vi "Ref.vi"() -> ()   [LabVIEW 2017]
uses:
  <vilib>/userdefined/High Color/IMAQdx.ctl
  <vilib>/myRIO/Common/Instrument Driver Framework/myRIO v1.0/UART/vis/myRIO v1.0 Close UART.vi
  LABVIEW2/colum_element.vi
  <vilib>/myRIO/Common/Instrument Driver Framework/Utilities/vis/FPGA Ref Manager.vi
  <vilib>/myRIO/Common/Instrument Driver Framework/myRIO v1.0/myRIO v1.0 Reset FPGA.vi
  <vilib>/myRIO/Common/Instrument Driver Framework/myRIO v1.0/IRQ/vis/myRIO v1.0 IRQ Info FGV.vi
  <vilib>/myRIO/Common/Instrument Driver Framework/myRIO v1.0/IRQ/vis/myRIO v1.0 Timer IRQ Info FGV.vi
  <vilib>/myRIO/Common/Instrument Driver Framework/myRIO v1.0/IRQ/vis/myRIO v1.0 ISR Agent.vi
  <vilib>/vision/driver/NI_Vision_Acquisition_Software.lvlib
  <vilib>/myRIO/Instrument Drivers/Utilities/Utilities.lvlib
  <vilib>/vision/NI_Vision_Development_Module.lvlib
panel:
  out "Numeric":i32
  out "Column_VALUE":i32
  out "Image Pixels (U8)":u8[][](array[numeric])
  in  "Optional Rectangle":i32[](array[numeric])=[0, 0, 640, 480]
  out "Threshold Image":T1(plugin-control)
  in  "Manual":cluster{sgl, sgl}(slide)={100.0, 255.0} caption="Threshold Range" scale=0.0..255.0
  in  "Stop":bool
  out "Image Preview":T1(plugin-control)
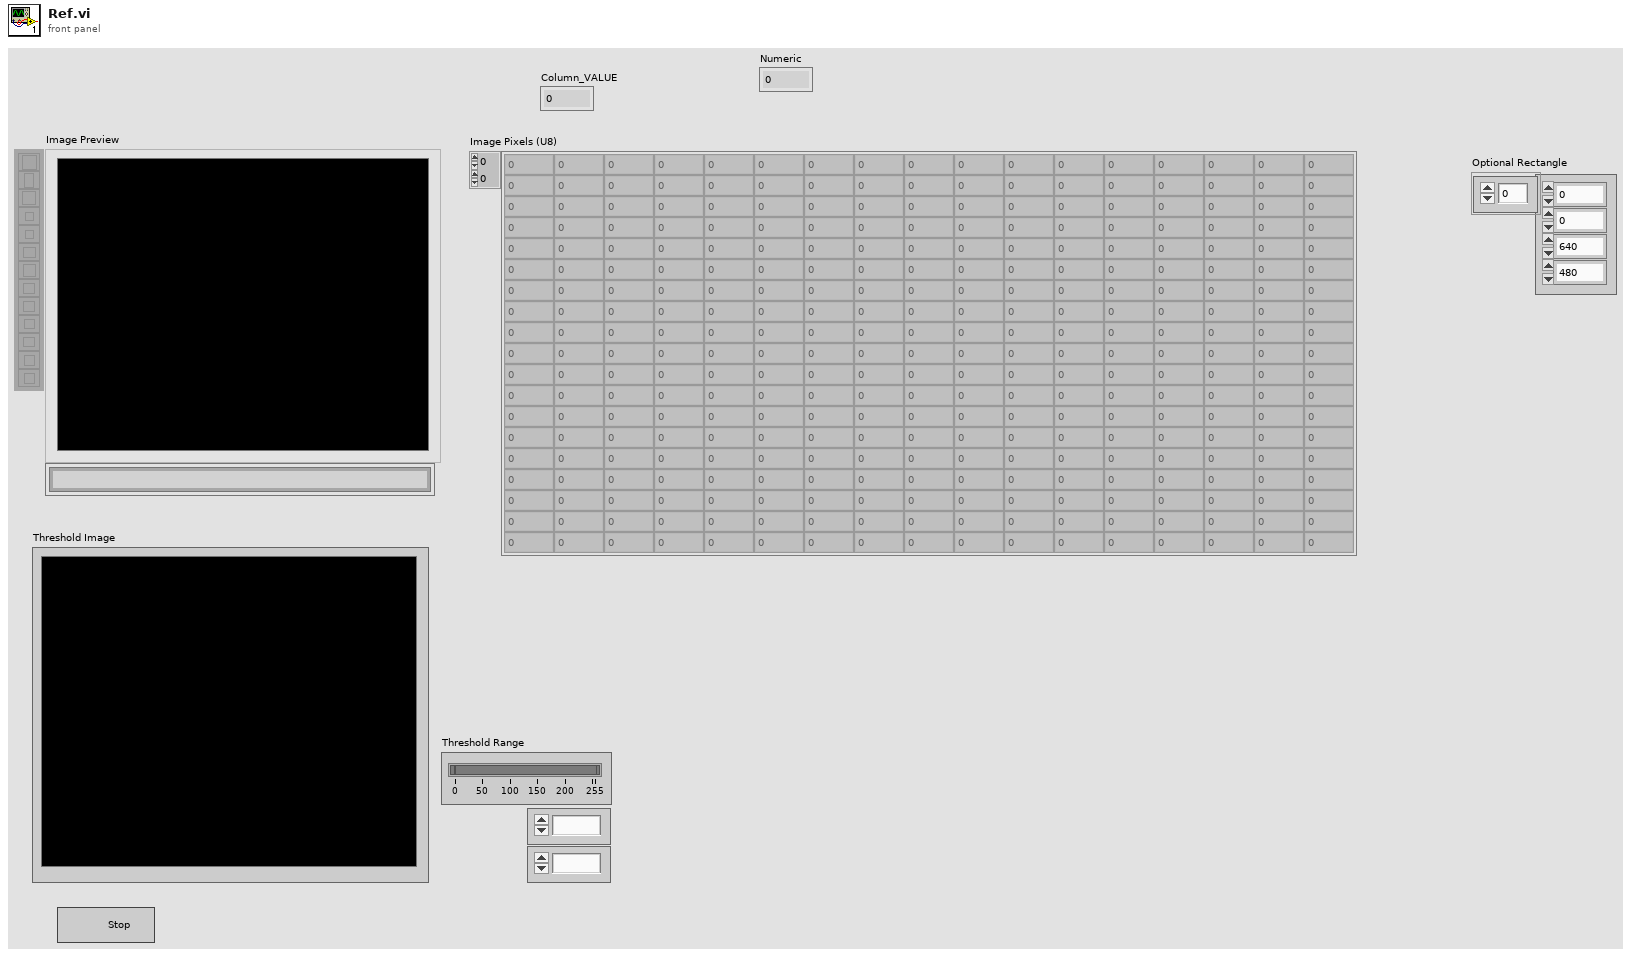
[diagram p1: front panel]
types:
  T1 = typedef "IMAQ Image.ctl" = refnum<image>
  T2 = typedef "IMAQdx.ctl" = refnum<k21>
  T3 = typedef "Image Type" = u32
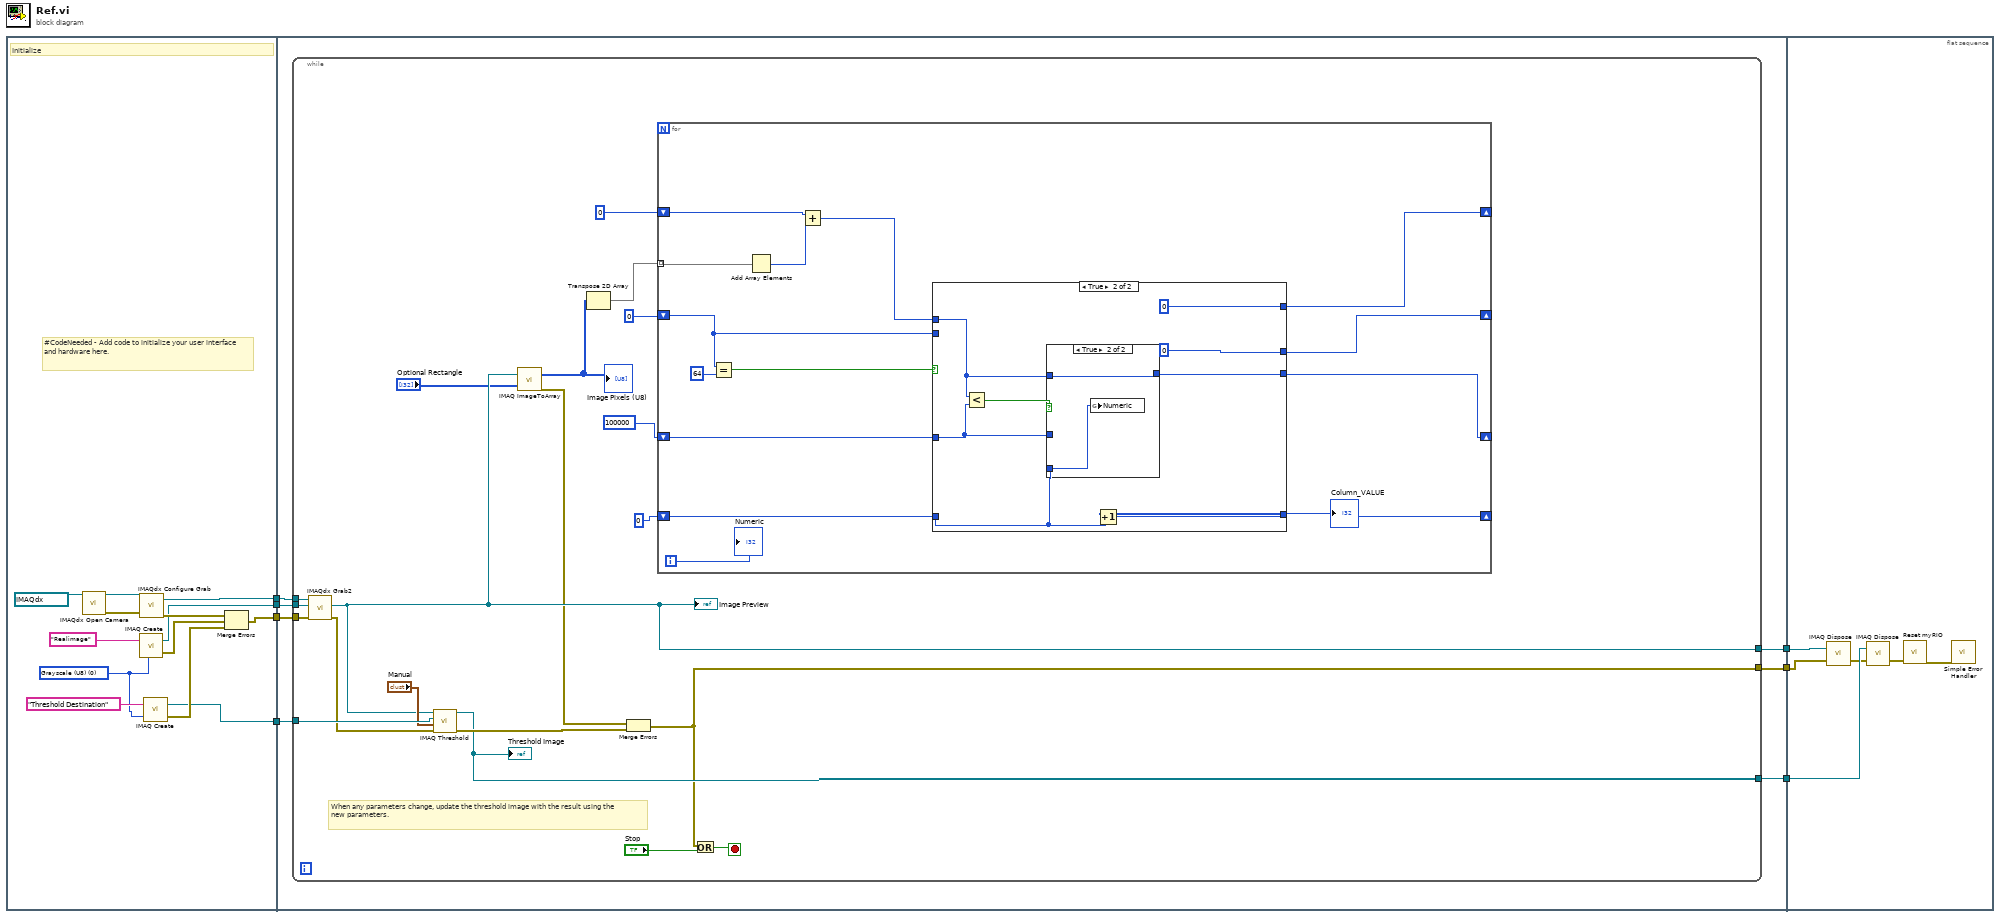
[diagram p0: block diagram]
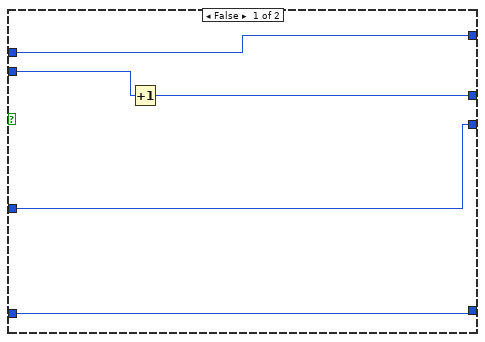
[diagram p2: hidden frame]
diagram:
  n1 = flat-sequence {
    tunnel: [w14] -> w7
    tunnel: [w13] -> w6
    tunnel: [w12] -> w5
    tunnel: [w8] -> w2
    tunnel: w7 -> [w27]
    tunnel: w6 -> [w26]
    tunnel: w5 -> [w25]
    tunnel: [w24] -> w4
    tunnel: [w23] -> w3
    tunnel: w2 -> [w22]
    tunnel: [w21] -> w1
    tunnel: w4 -> [w83]
    tunnel: w3 -> [w82]
    tunnel: w1 -> [w79]
    frame #0 {
      w10 = T3 0 items=["Grayscale (U8)", "Grayscale (I16)", "Grayscale (SGL)", "Complex (CSG)", "RGB (U32)", "HSL (U32)", "RGB (U64)", "Grayscale (U16)"] ("Image Type")
      # "#CodeNeeded - Add code to initialize your user interface and hardware here."
      # "Initialize"
      n2 = call <vilib>:"IMAQdx Open Camera.vi"("Session In"=T2 "cam0") -> ("error out"=w19:errorcluster, "Session Out"=w20:T2)  [unwired: 9 in]
      n3 = call "IMAQ Create"("Image Name"="Realimage", "Image Type"=w10) -> ("New Image"=w13:T1, "error out"=w16:errorcluster)  [unwired: 3 in]
      n4 = call <vilib>:"IMAQdx Configure Grab.vi"("error in"=w19, "Session In"=w20) -> ("error out"=w15:errorcluster, "Session Out"=w12:T2)  [unwired: 8 in]
      n5 = call "IMAQ Create"("Image Name"="Threshold Destination", "Image Type"=w10) -> ("New Image"=w8:T1, "error out"=w9:errorcluster)  [unwired: 3 in]
      n6 = Merge Errors(w15, w16, w9) -> (w14:errorcluster)
    }
    frame #1 {
      n7 = while {
        tunnel: w27 -> [w47]
        tunnel: w26 -> [w46]
        tunnel: w25 -> [w45]
        tunnel: [w35] -> w23
        tunnel: [w37] -> w24
        tunnel: w22 -> [w44]
        tunnel: [w38] -> w21
        stop <- w42 stop-if-true
        # "When any parameters change, update the threshold image with the result using the new parameters."
        n8 = call <vilib>:"IMAQdx Grab2.vi"("error in"=w47, "Image In"=w46, "Session In"=w45) -> ("error out"=w41:errorcluster, "Image Out"=w37:T1)  [unwired: 5 in, 2 out]
        "Image Preview" <- w37
        n9 = call "IMAQ Threshold"("error in (no error)"=w41, "Range"="Manual", "Image Dst"=w44, "Image Src"=w37) -> ("error out"=w40:errorcluster, "Image Dst Out"=w38:T1)  [unwired: 6 in]
        "Threshold Image" <- w38
        n10 = call "IMAQ ImageToArray"("Optional Rectangle"="Optional Rectangle", "Image"=w37) -> ("error out"=w34:errorcluster, "Image Pixels (U8)"=w33:u8[][])  [unwired: 2 in, 3 out]
        "Image Pixels (U8)" <- w33
        n11 = Transpose 2D Array(2D array=w33) -> (transposed array=w32:u8[][])
        n12 = Merge Errors(w34, w40) -> (w35:errorcluster)
        n13 = for {
          tunnel: w32 -> [w61] mode=indexing
          shift-right: [w55] -> _
          shift-left: 0 -> [w56]
          shift-right: [w51] -> _
          shift-left: 0 -> [w59]
          shift-right: [w53] -> _
          shift-left: 0 -> [w54]
          shift-right: [w48] -> _
          shift-left: 100000 -> [w49]
          i -> [w50]
          n14 = Equal?(x=w56, y=64) -> (x = y?=w57:bool)
          n15 = Add Array Elements(numeric array=w61) -> (sum=w60:u8)
          n16 = Add(x=w59, y=w60) -> (x+y=w52:i32)
          n17 = case shown="True" w57 {
            tunnel: w56 -> [w66 _]
            tunnel: [w65 0] -> w55
            tunnel: w54 -> [w64 w70]
            tunnel: [w64 w73] -> w53
            tunnel: w52 -> [w63 w69]
            tunnel: [w63 0] -> w51
            tunnel: w49 -> [w62 w67]
            tunnel: [w62 w68] -> w48
            frame False {
              n18 = Increment(x=w66) -> (x+1=w65:i32)
            }
            frame True {
              n19 = Less?(x=w69, y=w67) -> (x < y?=w71:bool)
              n20 = case shown="True" w71 {
                tunnel: w70 -> [_ w77]
                tunnel: w69 -> [_ w76]
                tunnel: [w75 w76] -> w68
                tunnel: w67 -> [w75 _]
                frame False {
                }
                frame True {
                  n21 = global write "colum_element.vi" "Numeric"(w77) -> ()
                }
              }
              n22 = Increment(x=w70) -> (x+1=w73:i32)
            }
          }
          "Column_VALUE" <- w53
          "Numeric" <- w50
        }
        n23 = Or(x=w35, y="Stop") -> (x .or. y?=w42:bool)
      }
    }
    frame #2 {
      n24 = call "IMAQ Dispose"("Image"=w83, "error in (no error)"=w82) -> ("error out"=w78:errorcluster)  [unwired: 4 in]
      n25 = call "IMAQ Dispose"("Image"=w79, "error in (no error)"=w78) -> ("error out"=w80:errorcluster)  [unwired: 4 in]
      n26 = call <vilib>:"Reset myRIO.vi"("error in (no error)"=w80) -> ("error out"=w81:errorcluster)  [unwired: 10 in]
      n27 = call <vilib>:"Simple Error Handler.vi"("error in (no error)"=w81) -> ()  [unwired: 4 in, 5 out]
    }
  }
